vi "VmagSanitise.vi"(11 "RawVmagUVWCone":dbl[][](array[numeric]) caption="Raw\n   Vmag         U             V             W          Cone") -> (3 "NaNsanitisedVmagUVWCone":dbl[][](array[numeric]) caption="NaN-sanitised\n   Vmag          U               V              W        Cone")   [LabVIEW 2016]
doc: "Ensures if any one component is NaN, all components will be set to NaN"
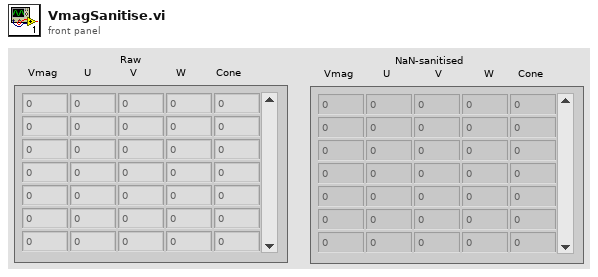
[diagram p1: front panel]
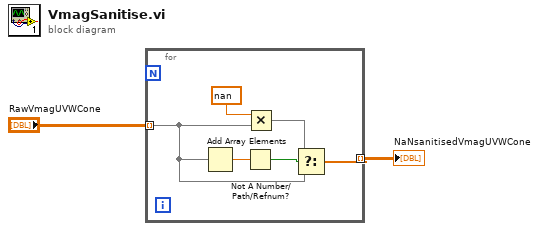
[diagram p0: block diagram]
diagram:
  n1 = for {
    tunnel: [w6] -> w2 mode=indexing
    tunnel: "RawVmagUVWCone" -> [w5] mode=indexing
    n2 = Add Array Elements(numeric array=w5) -> (sum=w8:dbl)
    n3 = Not A Number/Path/Refnum?(number/path/refnum=w8) -> (NaN/Path/Refnum?=w7:bool)
    n4 = Multiply(x=nan ("Numeric"), y=w5) -> (x*y=w4:dbl[])
    n5 = Select(t=w4, s=w7, f=w5) -> (s? t:f=w6:dbl[])
  }
  "NaNsanitisedVmagUVWCone" <- w2
